vi "Test CVT.vi"() -> ()   [LabVIEW 2014]
panel:
  out "data value":variant
  out "json cvt":string
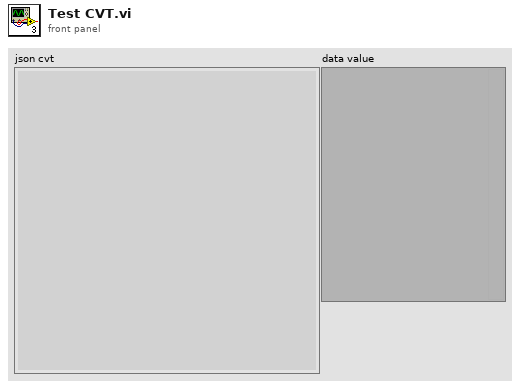
[diagram p1: front panel]
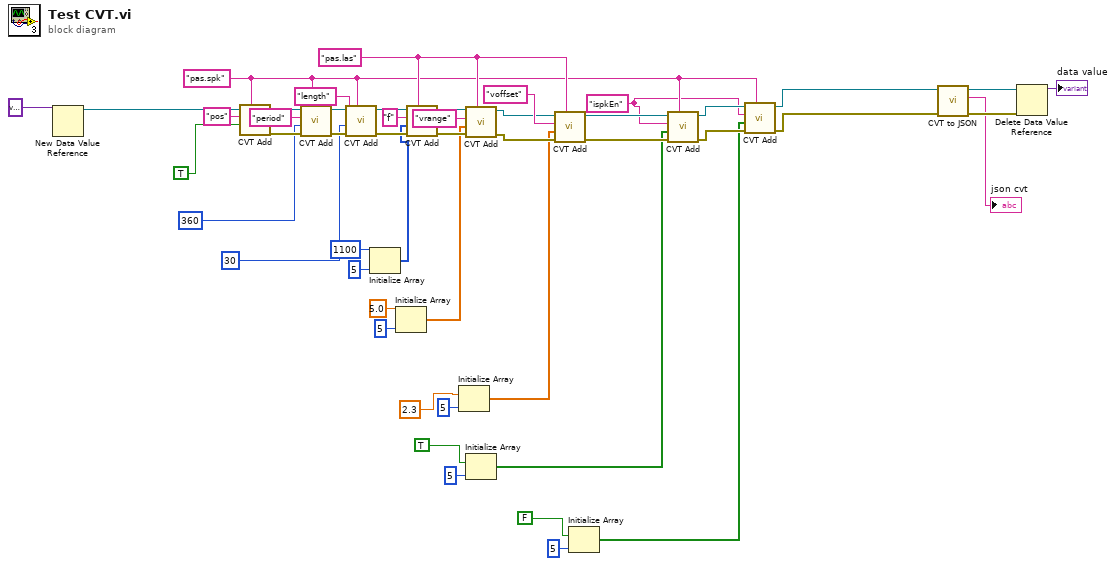
[diagram p0: block diagram]
diagram:
  w4 = "ispkEn" ("tag")
  w18 = "pas.las" ("Group")
  w5 = "pas.spk" ("Group")
  n1 = New Data Value Reference(data value=variant) -> (data value reference=w48:refnum<data-value>)  [unwired: 1 in, 1 out]
  n2 = call "CVT Add.vi"("Group"=w5, "Data"=TRUE, "tag"="pos", "cvt"=w48) -> ("error out"=w44:errorcluster, "cvt"=w45:refnum<data-value>)  [unwired: 6 in]
  n3 = call "CVT Add.vi"("Group"=w5, "error in"=w44, "Data"=360, "tag"="period", "cvt"=w45) -> ("error out"=w41:errorcluster, "cvt"=w40:refnum<data-value>)  [unwired: 5 in]
  n4 = call "CVT Add.vi"("Group"=w5, "error in"=w41, "Data"=30, "tag"="length", "cvt"=w40) -> ("error out"=w36:errorcluster, "cvt"=w37:refnum<data-value>)  [unwired: 5 in]
  n5 = Initialize Array(i16 1100 ("element"), 5 ("dimension size")) -> (w32:i16[])
  n6 = Initialize Array(5.0 ("element"), 5 ("dimension size")) -> (w26:dbl[])
  n7 = call "CVT Add.vi"("Group"=w18, "error in"=w36, "Data"=w32, "tag"="f", "cvt"=w37) -> ("error out"=w31:errorcluster, "cvt"=w30:refnum<data-value>)  [unwired: 5 in]
  n8 = Initialize Array(2.3 ("element"), 5 ("dimension size")) -> (w15:dbl[])
  n9 = call "CVT Add.vi"("Group"=w18, "error in"=w31, "Data"=w26, "tag"="vrange", "cvt"=w30) -> ("error out"=w19:errorcluster, "cvt"=w20:refnum<data-value>)  [unwired: 5 in]
  n10 = Initialize Array(TRUE, 5 ("dimension size")) -> (w10:bool[])
  n11 = call "CVT Add.vi"("Group"=w18, "error in"=w19, "Data"=w15, "tag"="voffset", "cvt"=w20) -> ("error out"=w13:errorcluster, "cvt"=w14:refnum<data-value>)  [unwired: 5 in]
  n12 = Initialize Array(FALSE, 5 ("dimension size")) -> (w1:bool[])
  n13 = call "CVT Add.vi"("Group"=w5, "error in"=w13, "Data"=w10, "tag"=w4, "cvt"=w14) -> ("error out"=w8:errorcluster, "cvt"=w9:refnum<data-value>)  [unwired: 5 in]
  n14 = call "CVT Add.vi"("Group"=w5, "error in"=w8, "Data"=w1, "tag"=w4, "cvt"=w9) -> ("error out"=w6:errorcluster, "cvt"=w7:refnum<data-value>)  [unwired: 5 in]
  n15 = call "CVT to JSON.vi"("error in"=w6, "cvt"=w7) -> ("error out"=w24:errorcluster, "json cvt"=→"json cvt":string, "cvt 2"=w25:refnum<data-value>)  [unwired: 7 in]
  n16 = Delete Data Value Reference(data value reference=w25, error in=w24) -> (data value=→"data value":variant)  [unwired: 1 out]
